vi "Configure Reference Channel (Others).vi"(0 "VISA resource name":refnum<visa-resource-name>, 1 "Auto Sweep Time (T: Enable)":bool=TRUE, 5 "Device Mode (1: BTS)":i32(ring)=1 items=["BTS"=1, "MS"=2], 7 "Channel Integration Bandwidth (3.84E+6 Hz)":dbl=3840000.0 format="%#.6g", 9 "Channel Span (5E+6 Hz)":dbl=5000000.0 format="%#.6g", 11 "error in (no error)":errorcluster, 12 "Manual Sweep Time (0.0663 s)":dbl=0.0663) -> (4 "VISA resource name out":refnum<visa-resource-name>, 15 "error out":errorcluster)   [LabVIEW 2018, in "Agilent MXA Series.lvlib"]
doc: "Configures the Channel Intergration Bandwidth, Channel Span and Sweep Time of the Reference Channel in Spectrum Emission Mask measurement."
uses:
  Agilent MXA Series.lvlib
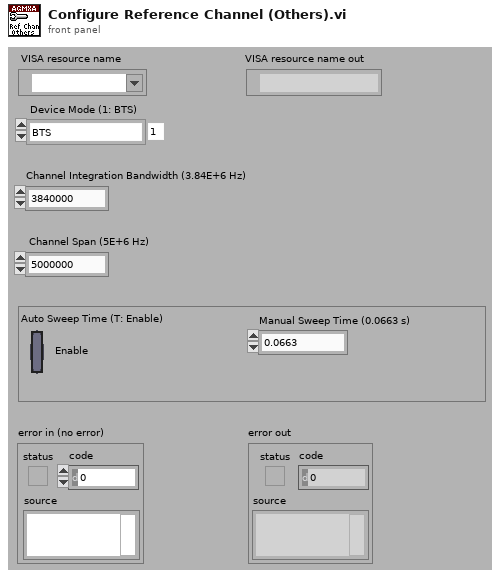
[diagram p1: front panel]
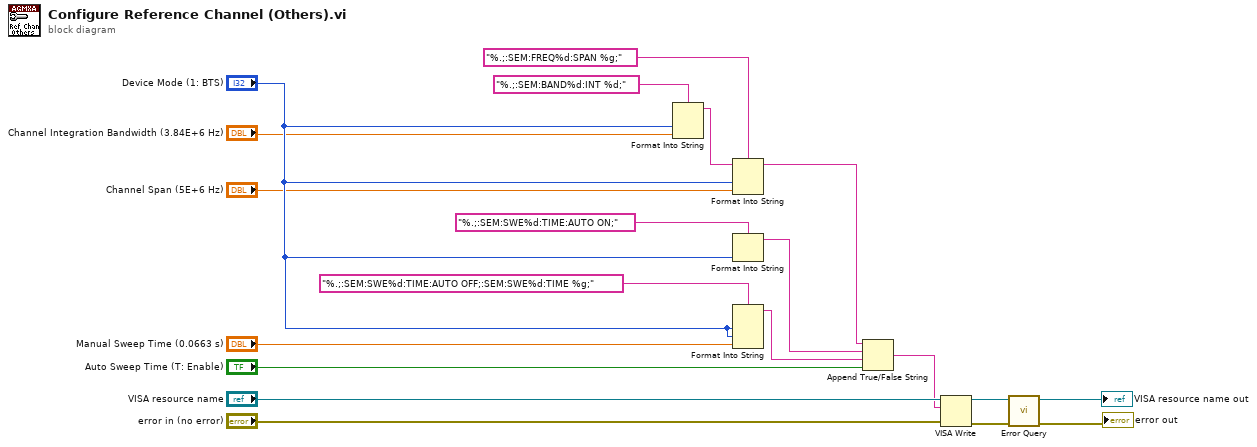
[diagram p0: block diagram]
diagram:
  n1 = Format Into String(format string="%.;:SEM:BAND%d:INT %d;" ("initial string"), "Device Mode (1: BTS)", "Channel Integration Bandwidth (3.84E+6 Hz)") -> (resulting string=w7:string)  [unwired: 2 in, 1 out]
  n2 = Format Into String(format string="%.;:SEM:FREQ%d:SPAN %g;" ("initial string"), initial string=w7, "Device Mode (1: BTS)", "Channel Span (5E+6 Hz)") -> (resulting string=w1:string)  [unwired: 1 in, 1 out]
  n3 = Format Into String(format string="%.;:SEM:SWE%d:TIME:AUTO ON;", "Device Mode (1: BTS)") -> (resulting string=w5:string)  [unwired: 2 in, 1 out]
  n4 = Format Into String(format string="%.;:SEM:SWE%d:TIME:AUTO OFF;:SEM:SWE%d:TIME %g;" ("initial string"), "Device Mode (1: BTS)", "Device Mode (1: BTS)", "Manual Sweep Time (0.0663 s)") -> (resulting string=w4:string)  [unwired: 2 in, 1 out]
  n5 = Append True/False String(1:"Auto Sweep Time (T: Enable)", 2:w4, 3:w5, 4:w1) -> (0:w2:string)
  n6 = VISA Write(VISA resource name="VISA resource name", write buffer=w2, error in (no error)="error in (no error)") -> (VISA resource name out=w15:refnum<visa-resource-name>, error out=w16:errorcluster)  [unwired: 1 out]
  n7 = call "Error Query.vi"("error in (no error)"=w16, "VISA resource name"=w15) -> ("error out"=→"error out":errorcluster, "VISA resource name out"=→"VISA resource name out":refnum<visa-resource-name>)  [unwired: 6 in, 2 out]
